vi "DSPMemory.vi"() -> ()   [LabVIEW 2014]
panel:
  out "Error":bool
  out "Value Read hex":i32 format="%.0x"
  in  "Value to Write":i32 min=0
  in  "Write":bool
  in  "Exit":bool
  in  "Read":bool
  in  "Type":enum16{"X", "Y", "P", "R", "D"}(ring)=enum."Y"
  in  "Board":T1(ring)=enum."TIMING_BOARD"
  out "Value Read":i32
  in  "Address":i32 min=0 format="%.0x"
  # "(hex)"
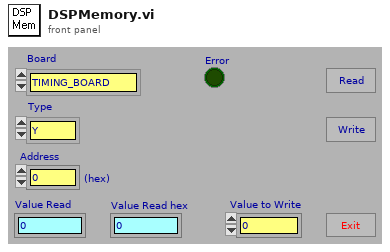
[diagram p1: front panel]
types:
  T1 = enum16{"not used", "PCI_BOARD", "TIMING_BOARD", "UTILITY_BOARD"}
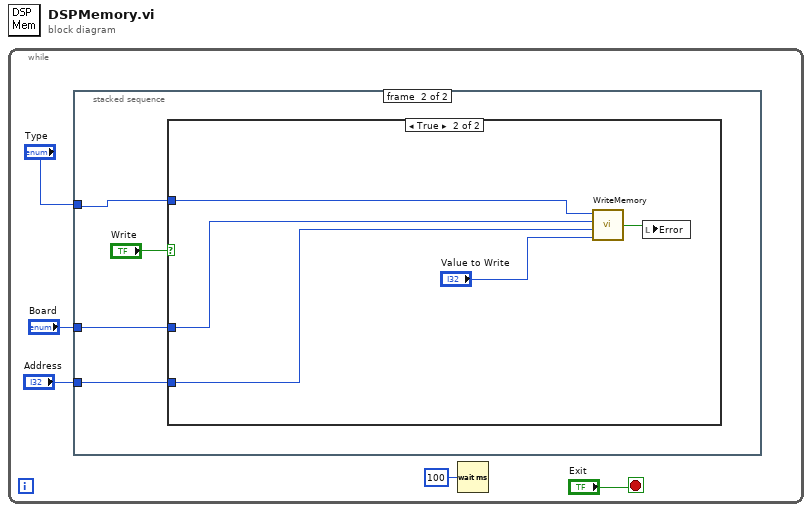
[diagram p0: block diagram]
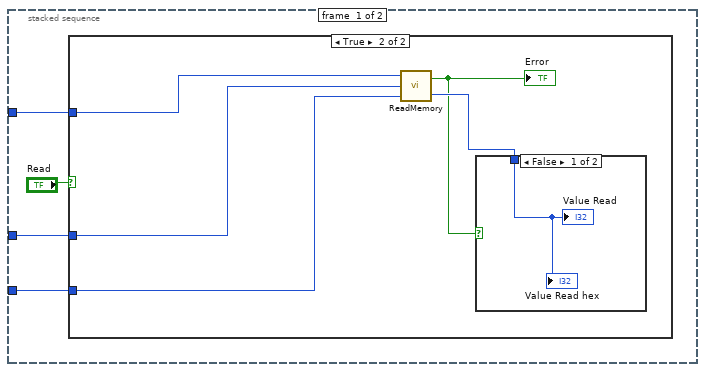
[diagram p2: hidden frame]
diagram:
  n1 = while {
    stop <- "Exit" stop-if-true
    n2 = stacked-sequence {
      tunnel: "Type" -> [w9 w19]
      tunnel: "Board" -> [w8 w18]
      tunnel: "Address" -> [w6 w17]
      frame #0 {
        n3 = case shown="True" "Read" {
          tunnel: w9 -> [_ w13]
          tunnel: w8 -> [_ w12]
          tunnel: w6 -> [_ w11]
          frame False {
          }
          frame True {
            n4 = call "ReadMemory.vi"("Address"=w11, "Board"=w12, "Type"=w13) -> ("Value"=w14:i32, "Error"=w10:bool)
            "Error" <- w10
            n5 = case shown="False" w10 {
              tunnel: w14 -> [w15 _]
              frame False {
                "Value Read" <- w15
                "Value Read hex" <- w15
              }
              frame True {
              }
            }
          }
        }
      }
      frame #1 {
        n6 = case shown="True" "Write" {
          tunnel: w19 -> [_ w24]
          tunnel: w18 -> [_ w23]
          tunnel: w17 -> [_ w22]
          frame False {
          }
          frame True {
            n7 = call "WriteMemory.vi"("Value"="Value to Write", "Address"=w22, "Board"=w23, "Type"=w24) -> ("Error"=w20:bool)
            n8 = local write "Error"(w20) -> ()
          }
        }
      }
    }
    n9 = Wait (ms)(milliseconds to wait=u32 100) -> ()  [unwired: 1 out]
  }
